vi "Set Sender.vi"(10 "Sender":refnum<class "Sender.lvclass">, 11 "Msg Strategy in":refnum<class "Msg Strategy.lvclass">) -> (3 "Msg Strategy out":refnum<class "Msg Strategy.lvclass">)   [LabVIEW 2021, in "jettl.lvlib" / "Msg Strategy.lvclass"]
uses:
  Msg Strategy.lvclass
  Sender/Sender/Sender.lvclass
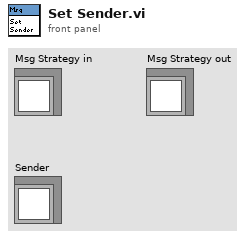
[diagram p1: front panel]
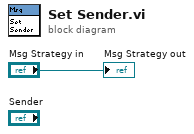
[diagram p0: block diagram]
diagram:
  "Msg Strategy out" <- "Msg Strategy in"
